vi "ConvertTimes - Array.vi"(1 "GP22 results":dbl[](array[numeric])) -> (0 "Array of times / s":dbl[](array[numeric]))   [LabVIEW 2014, in "GP22_TDC_Arduinoed.lvlib"]
doc: "Convert fixed point output of GP22 to time value in seconds."
uses:
  GP22_TDC_Arduinoed.lvlib
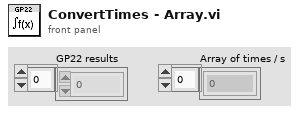
[diagram p1: front panel]
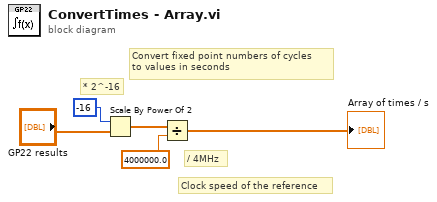
[diagram p0: block diagram]
diagram:
  # "Clock speed of the reference"
  # "Convert fixed point numbers of cycles\nto values in seconds"
  # "/ 4MHz"
  # "* 2^-16"
  n1 = Scale By Power Of 2(n=i16 -16, x="GP22 results") -> (x*2^n=w4:dbl[])
  n2 = Divide(x=w4, y=4000000.0) -> (x/y=→"Array of times / s":dbl[])
